vi "Actor Core.vi"(8 "error in":errorcluster, 11 "Nested in":refnum<class "QuickNoteUI.lvclass">) -> (0 "error out":errorcluster, 3 "Actor out":refnum<class "Actor.lvclass">)   [LabVIEW 2020, in "QuickNote.lvlib" / "QuickNoteUI.lvlib" / "QuickNoteUI.lvclass"]
doc: "(<B>Filename</B>: Actor Framework.lvlib:Actor.lvclass:Actor Core.vi)\n\nReceives messages to the actor, reacts to them, and initiates any error handling that may shut the actor down.\n\nDescendant classes may override this VI to append parallel tasks for the actor to complete while it handles messages. Overrides use the Call Parent Method node."
uses:
  QuickNoteUI.lvclass
  C:/Program Files/National Instruments/LabVIEW 2020/vi.lib/ActorFramework/Actor/Actor.lvclass
  <vilib>/ActorFramework/Actor/Actor.lvclass
  QuickNoteUI.lvclass/QuickNoteUI.ctl
  <vilib>/ActorFramework/Actor/Actor.lvclass/Actor.ctl
  <vilib>/ActorFramework/Message Enqueuer/Message Enqueuer.lvclass/Message Enqueuer.ctl
  <vilib>/ActorFramework/Message Enqueuer/Init from Existing Queue.vi
  <vilib>/ActorFramework/Message Enqueuer/Enqueue.vi
  <vilib>/ActorFramework/Stop Msg/Stop Msg.lvclass
  C:/Program Files/National Instruments/LabVIEW 2020/vi.lib/ActorFramework/Message/Message.lvclass
  <vilib>/ActorFramework/Message Priority Queue/Priority Enqueue.vi
  <vilib>/ActorFramework/Message Enqueuer/Message Enqueuer.lvclass
  Interface/DataGenerator Messages/BroadcastData Msg/BroadcastData Msg.lvclass
  Hardware Abstraction Layer/Component/Device/Device/DataExchange.ctl
  Interface/DataListener/DataListener.lvclass
panel:
  in  "SaveTemplate":bool
  in  "LoadTemplate":bool
  in  "QuickNote":string
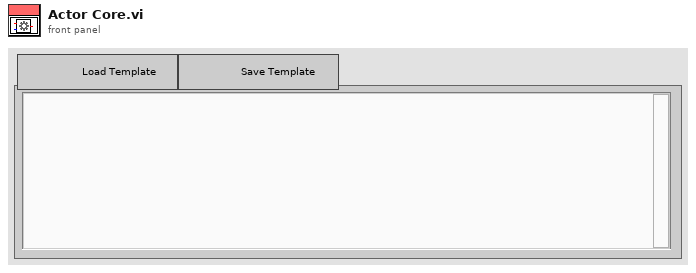
[diagram p1: front panel]
types:
  T1 = typedef "DataListener.lvclass/DataExchange.ctl" = cluster{"Source":string, "Target":string, "Type":string, "value":variant}
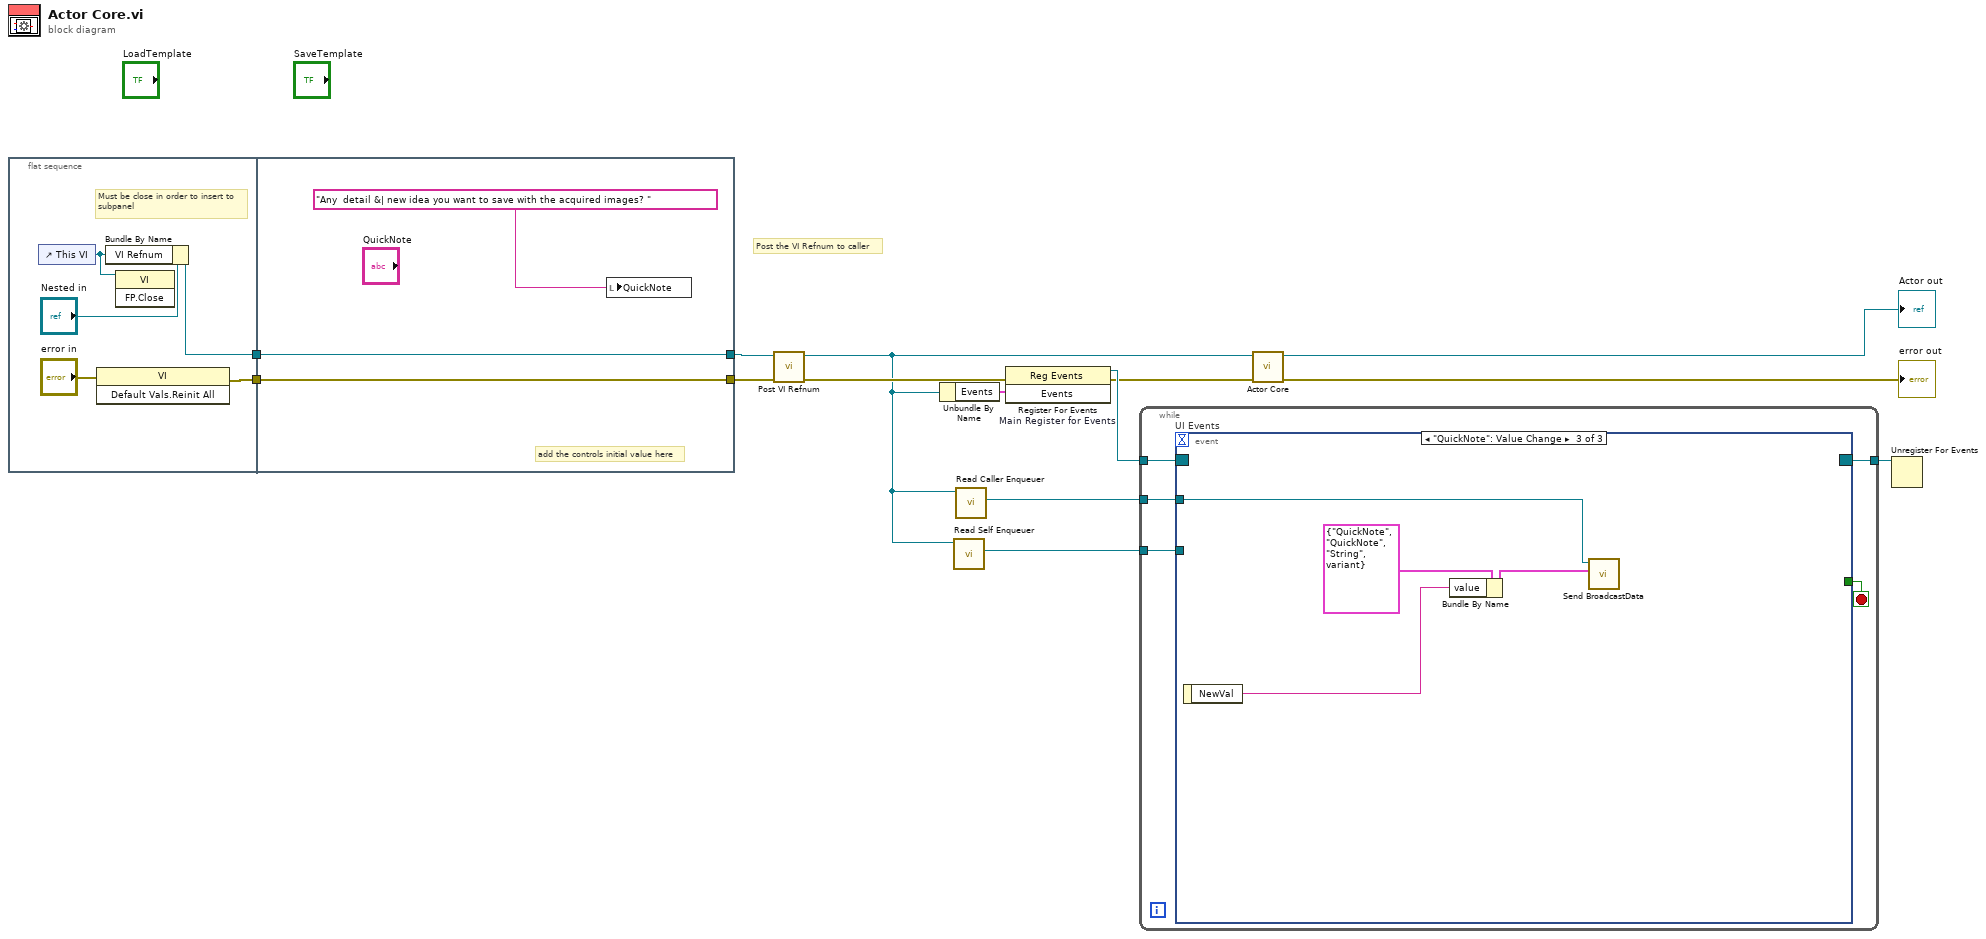
[diagram p0: block diagram]
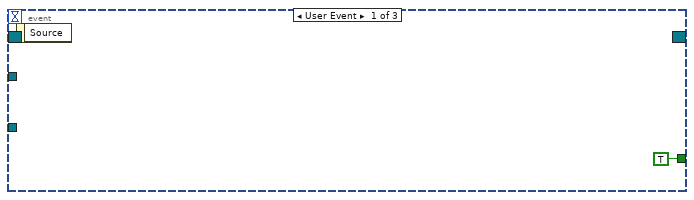
[diagram p2: hidden frame]
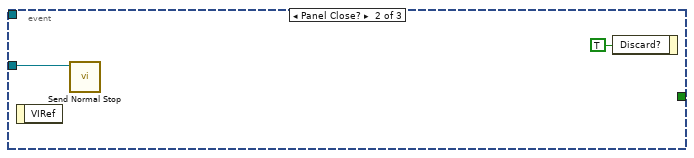
[diagram p3: hidden frame]
diagram:
  # "Post the VI Refnum to caller"
  n1 = flat-sequence {
    tunnel: [w17] -> w6
    tunnel: [w16] -> w5
    tunnel: [w21] -> w3
    tunnel: [w22] -> w7
    tunnel: w6 -> [w22]
    tunnel: w5 -> [w21]
    frame #0 {
      # "Must be close in order to insert to\nsubpanel"
      n2 = control-ref of="This VI"() -> (w15:refnum<vi>)
      n3 = invoke class="VI" method="Default Vals.Reinit All"(error in="error in") -> (error out=w17:errorcluster)  [unwired: 2 in, 2 out]
      n4 = Bundle By Name(cluster="Nested in", "VI Refnum"=w15) -> (w16:refnum<class "QuickNoteUI.lvclass">)
      n5 = invoke class="VI" method="FP.Close"(reference=w15) -> ()  [unwired: 2 in, 3 out]
    }
    frame #1 {
      # "add the controls initial value here"
      n6 = local write "QuickNote"("Any  detail &| new idea you want to save with the acquired images? " ("String")) -> ()
    }
  }
  n7 = call-dynamic "Post VI Refnum.vi"("error in (no error)"=w7, "Controller Template in"=w3) -> ("error out"=w4:errorcluster, "Controller Template out"=w2:refnum<class "QuickNoteUI.lvclass">)  [unwired: 8 in]
  n8 = Unbundle By Name(w2) -> ("Events"=w11:cluster{"Stop":refnum<user-event>})
  n9 = call <vilib>:"Read Self Enqueuer.vi"("Actor"=w2) -> ("Self Enqueuer"=w9:refnum<class "Message Enqueuer.lvclass">)  [unwired: 10 in]
  n10 = call <vilib>:"Read Caller Enqueuer.vi"("Actor"=w2) -> ("Caller Enqueuer"=w1:refnum<class "Message Enqueuer.lvclass">)  [unwired: 10 in]
  n11 = register-events "Main Register for Events"(error in=w4, w11) -> (reference out=w12:refnum<event-registration>, error out=w8:errorcluster)  [unwired: 1 in]
  n12 = while {
    tunnel: w12 -> [w27]
    tunnel: [w25] -> w10
    tunnel: w9 -> [w24]
    tunnel: w1 -> [w23]
    stop <- w26 stop-if-true
    n13 = event "UI Events" shown="[2] \"QuickNote\": Value Change" {
      selector: w27 -> [_ _ _]
      dyn-events: [_ _ _] -> w25
      timeout: _ -> [_ _ _]
      tunnel: [TRUE _ _] -> w26
      tunnel: w24 -> [_ w29 _]
      tunnel: w23 -> [_ _ w34]
      event User Event {
        n14 = event-data() -> ()  [unwired: 1 in, 1 out]
      }
      event Panel Close? {
        n15 = event-data() -> ()  [unwired: 1 in, 1 out]
        n16 = call <vilib>:"Send Normal Stop.vi"("Message Enqueuer"=w29) -> ()  [unwired: 10 in, 1 out]
        n17 = event-data("Discard?"=TRUE) -> ()  [unwired: 1 in, 1 out]
      }
      event "QuickNote": Value Change {
        n18 = event-data() -> ("NewVal"=w31:string)  [unwired: 1 in]
        n19 = Bundle By Name(cluster=T1 {"Source"="QuickNote", "Target"="QuickNote", "Type"="String", "value"=variant} ("DataExchange"), "value"=w31) -> (w32:T1)
        n20 = call "Send BroadcastData.vi"("DataExchange"=w32, "Message Enqueuer"=w34) -> ()  [unwired: 8 in, 2 out]
      }
    }
  }
  n21 = call-parent "Actor Core.vi"("error in"=w8, "Actor in"=w2) -> ("error out"=→"error out":errorcluster, "Actor out"=→"Actor out":refnum<class "Actor.lvclass">)  [unwired: 8 in]
  n22 = Unregister For Events(event registration refnum=w10) -> ()  [unwired: 1 in, 1 out]
